vi "metronome.vi"(1 "Start Time (ns)":u64, 2 "Loop Rate (ns)":u32=500) -> (0 "Finished late?":bool)   [LabVIEW 2011, in "EPS_Timekeeper.lvlib"]
uses:
  <vilib>/addons/Electrical Power/Example Support/PMU/Time Keeper/EPS_Timekeeper.lvlib
  <vilib>/addons/Electrical Power/Example Support/PMU/Time Keeper/timekeeper time (g).vi
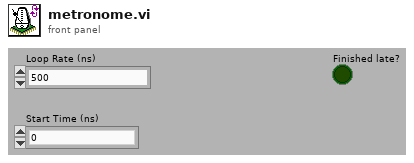
[diagram p1: front panel]
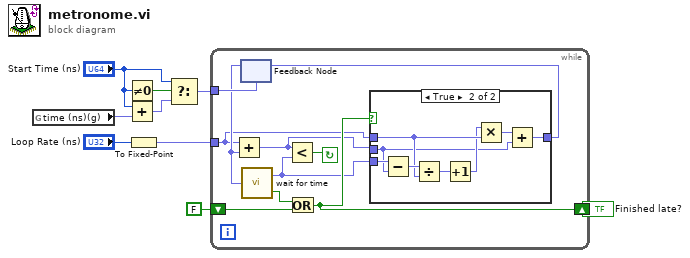
[diagram p0: block diagram]
diagram:
  n1 = global read "timekeeper time (g).vi" "time (ns)(g)"() -> (w2:fxp<+,64,64>)
  n2 = Not Equal To 0?(x="Start Time (ns)") -> (x != 0?=w6:bool)
  n3 = Add(x="Start Time (ns)", y=w2) -> (x+y=w5:fxp<+,64,64>)
  n4 = To Fixed-Point(number="Loop Rate (ns)") -> (fixed-point=w9:fxp<+,32,32>)  [unwired: 1 in]
  n5 = Select(t="Start Time (ns)", s=w6, f=w5) -> (s? t:f=w3:fxp<+,64,64>)
  n6 = while {
    tunnel: w9 -> [w13]
    tunnel: w3 -> [w19]
    shift-right: [w15] -> w8
    shift-left: FALSE ("Time already elapsed") -> [w16]
    stop <- w18 continue-if-true
    n7 = feedback #1(w19) -> (w14:fxp<+,64,64>)
    n8 = Add(x=w13, y=w14) -> (x+y=w12:fxp<+,64,64>)
    n9 = call <vilib>:"wait for time.vi"("Future Time (ns)"=w14) -> ("Time already elapsed"=w17:bool, "actual time (ns)"=w10:fxp<+,64,64>)
    n10 = Less?(x=w12, y=w10) -> (x < y?=w18:bool)
    n11 = Or(x=w17, y=w16) -> (x .or. y?=w15:bool)
    n12 = case shown="True" w15 {
      tunnel: w13 -> [_ w26]
      tunnel: w12 -> [w20 w22]
      tunnel: [w20 w21] -> w11
      tunnel: w10 -> [_ w28]
      frame False {
      }
      frame True {
        n13 = Subtract(x=w28, y=w22) -> (x-y=w27:fxp<+,64,64>)
        n14 = Divide(x=w27, y=w26) -> (x/y=w25:fxp<+,64,64>)
        n15 = Increment(x=w25) -> (x+1=w24:fxp<+,64,64>)
        n16 = Multiply(x=w24, y=w26) -> (x*y=w23:fxp<+,64,64>)
        n17 = Add(x=w23, y=w22) -> (x+y=w21:fxp<+,64,64>)
      }
    }
    n18 = feedback-in #1(w11) -> ()
  }
  "Finished late?" <- w8
